vi "MathDegToRad.vi"(11 "Deg":dbl) -> (3 "Rad":dbl)   [LabVIEW 2014]
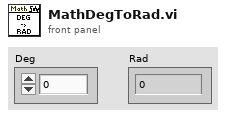
[diagram p1: front panel]
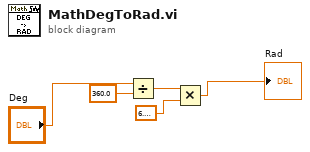
[diagram p0: block diagram]
diagram:
  n1 = Divide(x="Deg", y=360.0) -> (x/y=w3:dbl)
  n2 = Multiply(x=w3, y=6.283185307179586) -> (x*y=→"Rad":dbl)
